vi "Notify Monitor.vi"(8 "error in (no error)":errorcluster, 11 "Monitored Actor in":refnum<class "Monitored Actor.lvclass">) -> (0 "error out":errorcluster, 3 "Monitored Actor out":refnum<class "Monitored Actor.lvclass">)   [LabVIEW 2023, in "Monitored Actor.lvlib" / "Monitored Actor.lvclass"]
doc: "Notifies the actor monitor that a new actor has spawned\n\nCopyright: MGI 2016\nAuthor: Derek Trepanier"
uses:
  Library/Monitored Actor.lvclass
  C:/Users/Public/Documents/Development/builds/Framework/Actor Framework.lvlibp/1abvi3w/vi.lib/ActorFramework/Actor/Actor.lvclass
  Library/Monitored Actor.lvclass/Monitored Actor.ctl
  Actor Monitor/Actor Monitor Messages/Actor Launched Msg/Actor Launched Msg.lvclass
  Actor Monitor/Actor Monitor Messages/Update Label Msg/Update Label Msg.lvclass
  builds/Framework/Actor Framework.lvlibp/1abvi3w/vi.lib/ActorFramework/Actor/Actor.lvclass
  builds/Framework/Actor Framework.lvlibp/1abvi3w/vi.lib/ActorFramework/Message Enqueuer/Message Enqueuer.lvclass
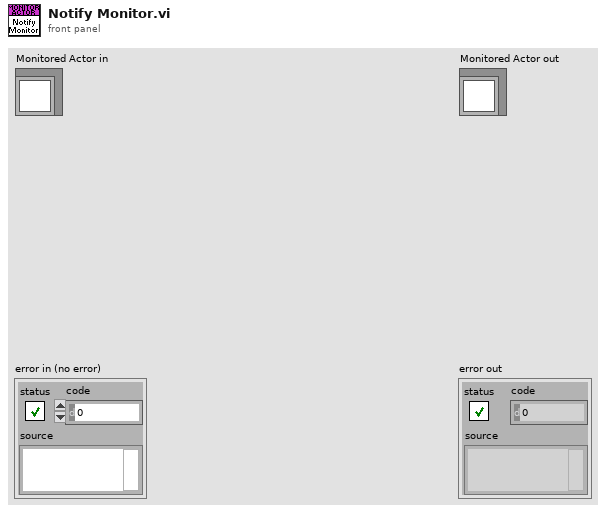
[diagram p1: front panel]
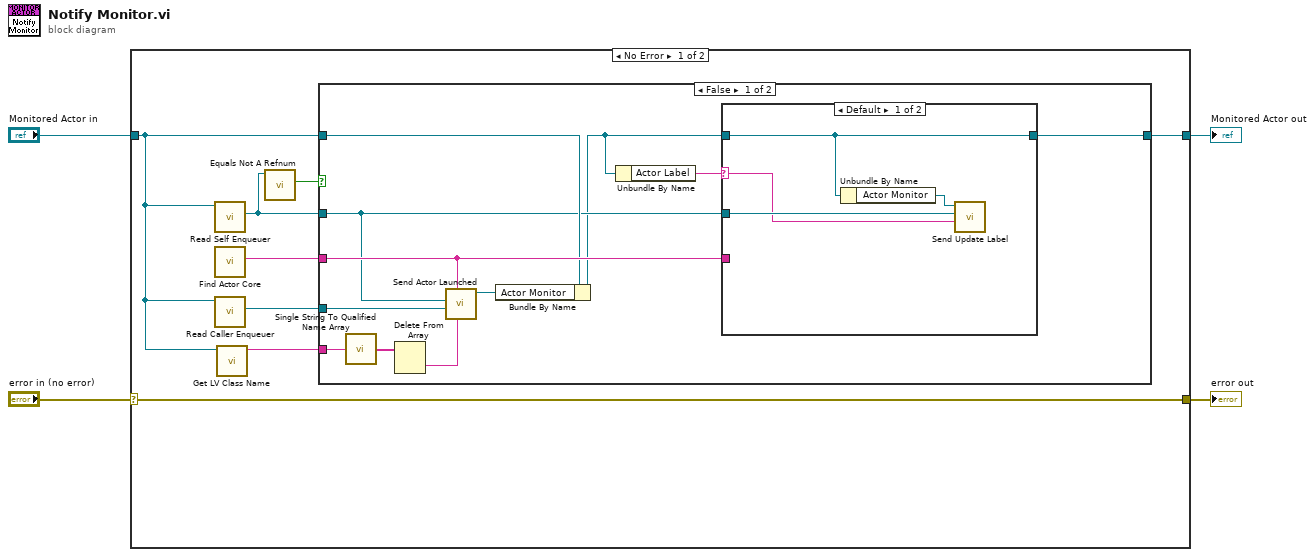
[diagram p0: block diagram]
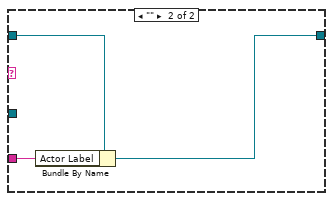
[diagram p2: hidden frame]
diagram:
  n1 = case shown="No Error" "error in (no error)" {
    selector: "error in (no error)" -> [w5 w33]
    tunnel: [w5 w33] -> w3
    tunnel: [w11 w32] -> w1
    tunnel: "Monitored Actor in" -> [w9 w32]
    frame No Error {
      n2 = call "Read Self Enqueuer.vi"("Actor"=w9) -> ("Self Enqueuer"=w7:refnum<class "Message Enqueuer.lvclass">)  [unwired: 10 in]
      n3 = call "Find Actor Core.vi"() -> ("Actor Core VI Name"=w10:string)  [unwired: 10 in, 1 out]
      n4 = call "Read Caller Enqueuer.vi"("Actor"=w9) -> ("Caller Enqueuer"=w12:refnum<class "Message Enqueuer.lvclass">)  [unwired: 10 in]
      n5 = call <vilib>:"Get LV Class Name.vi"("object"=w9) -> ("class name"=w8:string)  [unwired: 9 in, 1 out]
      n6 = call "Equals Not A Refnum.vi"("Message Enqueuer"=w7) -> ("Not a refnum?"=w6:bool)  [unwired: 10 in]
      n7 = case shown="False" w6 {
        tunnel: w12 -> [w23 _]
        tunnel: [w22 w31] -> w11
        tunnel: w10 -> [w20 _]
        tunnel: w9 -> [w19 w31]
        tunnel: w8 -> [w17 _]
        tunnel: w7 -> [w18 _]
        frame False {
          n8 = call <vilib>:"Single String To Qualified Name Array.vi"("Fully Qualified String"=w17) -> ("Fully Qualified Array"=w16:string[])
          n9 = Delete From Array(array=w16) -> (deleted portion=w15:string)  [unwired: 2 in, 1 out]
          n10 = call "Send Actor Launched.vi"("Actor Type"=w15, "Actor Core VI"=w20, "Actor's Caller Q"=w23, "Actor's Self Q"=w18) -> ("Message Enqueuer out"=w13:refnum<class "Message Enqueuer.lvclass">)  [unwired: 6 in, 1 out]
          n11 = Bundle By Name(cluster=w19, "Actor Monitor"=w13) -> (w14:refnum<class "Monitored Actor.lvclass">)
          n12 = Unbundle By Name(w14) -> ("Actor Label"=w21:string)
          n13 = case shown="Default" w21 {
            selector: w21 -> [w26 _]
            tunnel: w14 -> [w25 w30]
            tunnel: w18 -> [w27 _]
            tunnel: [w25 w29] -> w22
            tunnel: w20 -> [_ w28]
            frame Default {
              n14 = Unbundle By Name(w25) -> ("Actor Monitor"=w24:refnum<class "Message Enqueuer.lvclass">)
              n15 = call "Send Update Label.vi"("Actor's Label"=w26, "Actor's Self Q"=w27, "Message Enqueuer in"=w24) -> ()  [unwired: 7 in, 2 out]
            }
            frame "" {
              n16 = Bundle By Name(cluster=w30, "Actor Label"=w28) -> (w29:refnum<class "Monitored Actor.lvclass">)
            }
          }
        }
        frame True {
        }
      }
    }
    frame Error {
    }
  }
  "error out" <- w3
  "Monitored Actor out" <- w1
